vi "Set SCIP Mode.vi"(8 "error in (no error)":errorcluster, 10 "Protocol (2: SCIP 2.0)":u32(ring)=2 items=["Convert to Latest", "SCIP 1.1", "SCIP 2.0", "SCIP 2.2"], 11 "VISA resource name":refnum<visa-resource-name>) -> (0 "error out":errorcluster, 3 "VISA resource name out":refnum<visa-resource-name>)   [LabVIEW 2014, in "Hokuyo URG Series.lvlib"]
doc: "Sets a SCIP 1.1 instrument to use the SCIP 2.0 protocol. Not all instruments or firmware revisions support this call. Refer to the instrument manual for more informaiton. This VI is called from the initialization VI and should generally not be called on its own."
uses:
  Hokuyo URG Series.lvlib
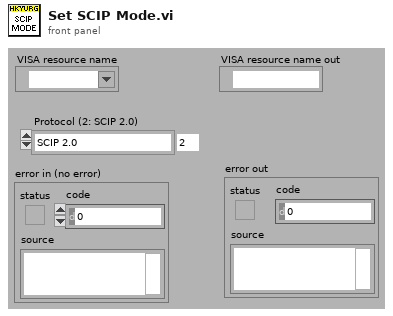
[diagram p1: front panel]
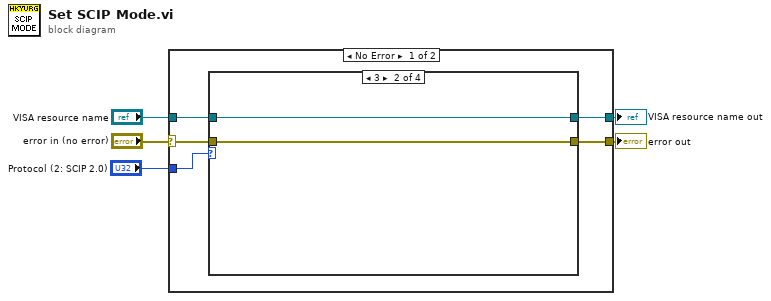
[diagram p0: block diagram]
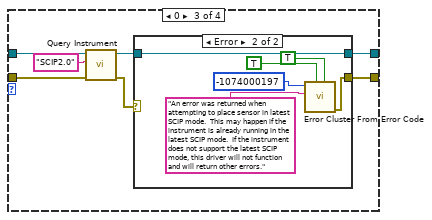
[diagram p3: hidden frame]
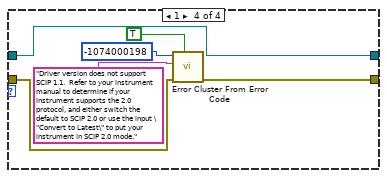
[diagram p5: hidden frame]
diagram:
  n1 = case shown="No Error" "error in (no error)" {
    selector: "error in (no error)" -> [w6 w36]
    tunnel: [w10 w36] -> w5
    tunnel: [w9 w37] -> w4
    tunnel: "VISA resource name" -> [w8 w37]
    tunnel: "Protocol (2: SCIP 2.0)" -> [w7 _]
    frame No Error {
      n2 = case shown="3" w7 {
        tunnel: w8 -> [w12 w14 w20 w34]
        tunnel: [w12 w14 w16 w34] -> w9
        tunnel: w6 -> [w11 w13 w19 w31]
        tunnel: [w11 w13 w15 w35] -> w10
        frame 2, Default {
        }
        frame 3 {
        }
        frame 0 {
          n3 = call "Query Instrument.vi"("error in"=w19, "Command"="SCIP2.0" ("Change to SCIP 2.0"), "VISA Resource Name"=w20) -> ("error out"=w18:errorcluster, "VISA Resource Name Out"=w17:refnum<visa-resource-name>)  [unwired: 6 in, 1 out]
          n4 = case shown="Error" w18 {
            selector: w18 -> [w22 _]
            tunnel: w17 -> [w23 w26]
            tunnel: [w23 w26] -> w16
            tunnel: [w22 w24] -> w15
            frame No Error {
            }
            frame Error {
              n5 = call <vilib>:"Error Cluster From Error Code.vi"("is warning? (False)"=TRUE, "show call chain? (False)"=TRUE, "error message (\"\")"="An error was returned when attempting to place sensor in latest SCIP mode.  This may happen if the instrument is already running in the latest SCIP mode.  If the instrument does not support the latest SCIP mode, this driver will not function and will return other errors." ("error message (\"\")"), "error code (0)"=-1074000197) -> ("error out"=w24:errorcluster)  [unwired: 5 in]
            }
          }
        }
        frame 1 {
          n6 = call <vilib>:"Error Cluster From Error Code.vi"("show call chain? (False)"=TRUE, "error in (no error)"=w31, "error message (\"\")"="Driver version does not support SCIP 1.1.  Refer to your instrument manual to determine if your instrument supports the 2.0 protocol, and either switch the default to SCIP 2.0 or use the input \"Convert to Latest\" to put your instrument in SCIP 2.0 mode." ("error message (\"\")"), "error code (0)"=-1074000198) -> ("error out"=w35:errorcluster)  [unwired: 5 in]
        }
      }
    }
    frame Error {
    }
  }
  "error out" <- w5
  "VISA resource name out" <- w4
